vi "Dynamic call-general.vi"(8 "error in (no error)":errorcluster, 11 "vi path":path) -> (0 "error out":errorcluster)   [LabVIEW 2020]
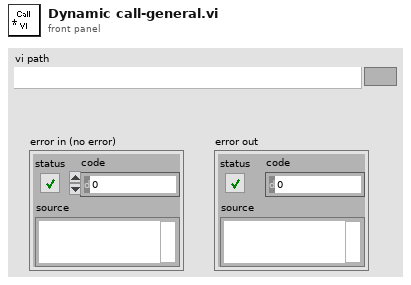
[diagram p1: front panel]
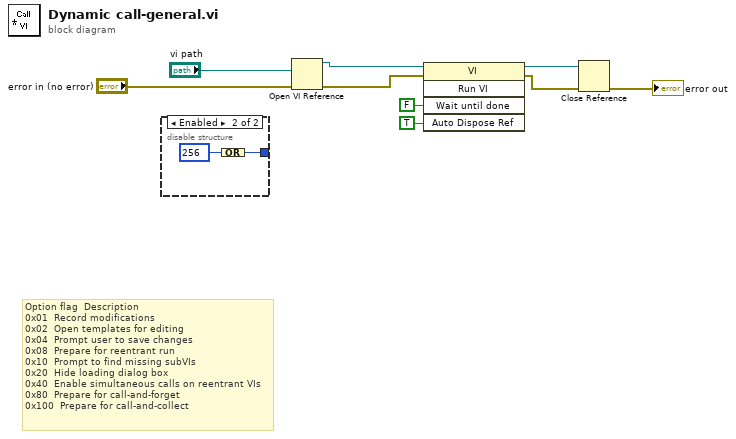
[diagram p0: block diagram]
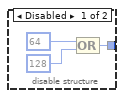
[diagram p2: hidden frame]
diagram:
  # "Option flag \tDescription\n0x01 \tRecord modifications\n0x02 \tOpen templates for editing\n0x04 \tPrompt user to save changes\n0x08 \tPrepare for reentrant run\n0x10 \tPrompt to find missing subVIs\n0x20 \tHide loading dialog box\n0x40 \tEnable simultaneous calls on reentrant VIs\n0x80 \tPrepare for call-and-forget\n0x100 \tPrepare for call-and-collect"
  n1 = disable-structure shown="Enabled" {
    disable-tunnel: [w12 w14] -> _
    frame Disabled {
      n2 = Compound Arithmetic op=OR(64, 128) -> (w12:i32)
    }
    frame Enabled {
      n3 = Compound Arithmetic op=OR(256) -> (w14:i32)
    }
  }
  n4 = Open VI Reference(vi path="vi path", error in (no error)="error in (no error)") -> (vi reference=w2:refnum<vi>, error out=w4:errorcluster)  [unwired: 4 in]
  n5 = invoke on="Invoke Node" class="VI" method="Run VI"(reference=w2, error in=w4, "Wait until done"=FALSE ("Wait Until Done"), "Auto Dispose Ref"=TRUE ("Auto Dispose Reference")) -> (reference out=w1:refnum<vi>, error out=w3:errorcluster)  [unwired: 1 in, 3 out]
  n6 = Close Reference(reference=w1, error in (no error)=w3) -> (error out=→"error out":errorcluster)
